vi "Package Must Exist.vi"(8 "error in (no error)":errorcluster, 11 "InitAction in":refnum<class "InitAction.lvclass">) -> (0 "error out":errorcluster, 2 "Pkg Must Exist":bool, 3 "InitAction out":refnum<class "InitAction.lvclass">)   [LabVIEW 2020, in "GPackTools.lvlib" / "InitAction.lvclass"]
uses:
  InitAction.lvclass
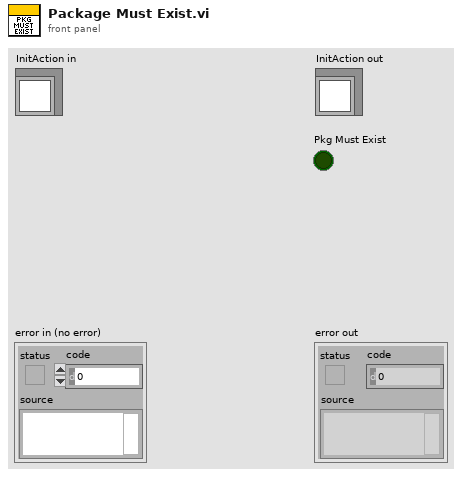
[diagram p1: front panel]
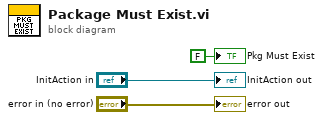
[diagram p0: block diagram]
diagram:
  "error out" <- "error in (no error)"
  "InitAction out" <- "InitAction in"
  "Pkg Must Exist" <- FALSE ("Pkg Must Exist")
